vi "TF to DBL Converstion (SubVI).vi"(0 "4_IN":bool, 1 "5_IN":bool, 2 "6_IN":bool, 3 "7_IN":bool, 4 "8_IN":bool, 5 "9_IN":bool, 6 "10_IN":bool, 7 "11_IN":bool, 8 "3_IN":bool, 9 "12_IN":bool, 10 "2_IN":bool, 11 "13_IN":bool, 12 "1_IN":bool, 13 "14_IN":bool) -> (14 "1_OUT":dbl, 15 "14_OUT":dbl, 16 "2_OUT":dbl, 17 "13_OUT":dbl, 18 "3_OUT":dbl, 19 "12_OUT":dbl, 20 "4_OUT":dbl, 21 "5_OUT":dbl, 22 "6_OUT":dbl, 23 "7_OUT":dbl, 24 "8_OUT":dbl, 25 "9_OUT":dbl, 26 "10_OUT":dbl, 27 "11_OUT":dbl)   [LabVIEW 2020]
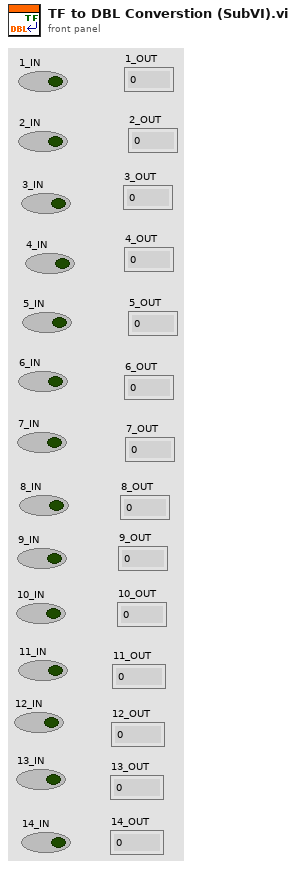
[diagram p1: front panel]
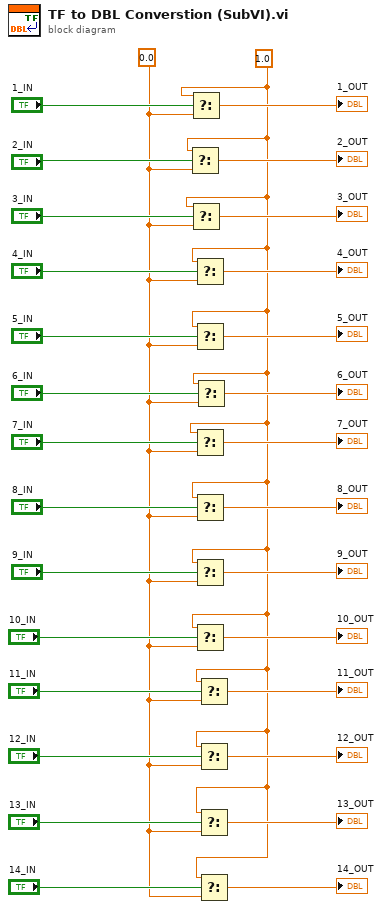
[diagram p0: block diagram]
diagram:
  w2 = 1.0 ("t")
  w1 = 0.0 ("t")
  n1 = Select(t=w2, s="2_IN", f=w1) -> (s? t:f=→"2_OUT":dbl)
  n2 = Select(t=w2, s="1_IN", f=w1) -> (s? t:f=→"1_OUT":dbl)
  n3 = Select(t=w2, s="3_IN", f=w1) -> (s? t:f=→"3_OUT":dbl)
  n4 = Select(t=w2, s="4_IN", f=w1) -> (s? t:f=→"4_OUT":dbl)
  n5 = Select(t=w2, s="5_IN", f=w1) -> (s? t:f=→"5_OUT":dbl)
  n6 = Select(t=w2, s="7_IN", f=w1) -> (s? t:f=→"7_OUT":dbl)
  n7 = Select(t=w2, s="8_IN", f=w1) -> (s? t:f=→"8_OUT":dbl)
  n8 = Select(t=w2, s="9_IN", f=w1) -> (s? t:f=→"9_OUT":dbl)
  n9 = Select(t=w2, s="10_IN", f=w1) -> (s? t:f=→"10_OUT":dbl)
  n10 = Select(t=w2, s="6_IN", f=w1) -> (s? t:f=→"6_OUT":dbl)
  n11 = Select(t=w2, s="11_IN", f=w1) -> (s? t:f=→"11_OUT":dbl)
  n12 = Select(t=w2, s="12_IN", f=w1) -> (s? t:f=→"12_OUT":dbl)
  n13 = Select(t=w2, s="13_IN", f=w1) -> (s? t:f=→"13_OUT":dbl)
  n14 = Select(t=w2, s="14_IN", f=w1) -> (s? t:f=→"14_OUT":dbl)
